vi "Test_PreloadNormalMsg_SendHighPriorityStop_StopImmediately.vi"(8 "error in (no error)":errorcluster, 11 "TestCase in":refnum<class "TestPriorityStopMessage.lvclass">) -> (0 "error out":errorcluster, 3 "TestCase out":refnum<class "TestPriorityStopMessage.lvclass">)   [LabVIEW 2017, in "TestPriorityStopMessage.lvclass"]
uses:
  TestPriorityStopMessage.lvclass
  <vilib>/ActorFramework/Message Enqueuer/Message Priority.ctl
  <vilib>/ActorFramework/Message Enqueuer/Message Enqueuer.lvclass/Message Enqueuer.ctl
  Doubles/MessageCountsExecutions/MessageCountsExecutions.lvclass
  C:/Program Files (x86)/National Instruments/LabVIEW 2017/vi.lib/ActorFramework/Message/Message.lvclass
  Doubles/ActorBlockedUntilNotified/ActorBlockedUntilNotified.lvclass
  C:/Program Files (x86)/National Instruments/LabVIEW 2017/vi.lib/ActorFramework/Actor/Actor.lvclass
  <vilib>/ActorFramework/Stop Msg/Stop Msg.lvclass
  <vilib>/ActorFramework/Message Priority Queue/Priority Enqueue.vi
  <vilib>/ActorFramework/Actor/Actor.lvclass
  <vilib>/ActorFramework/Message Enqueuer/Message Enqueuer.lvclass
  Source/PriorityStopMessage/PriorityStopMessage.lvclass
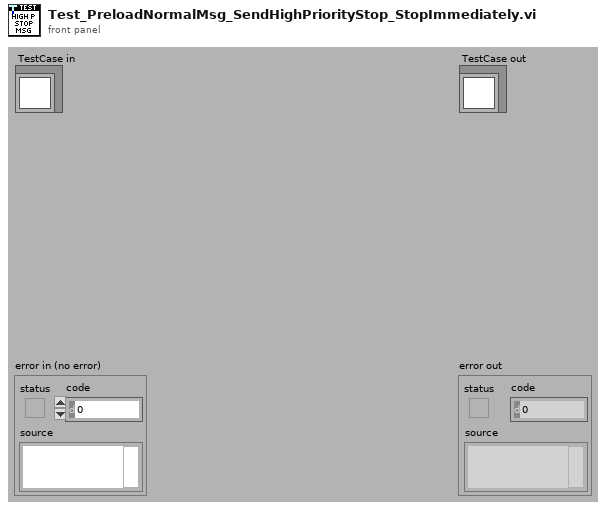
[diagram p1: front panel]
types:
  T1 = typedef "Actor Framework.lvlib/Message Enqueuer.lvclass/Message Priority.ctl" = enum16{"Low", "Normal", "High"}
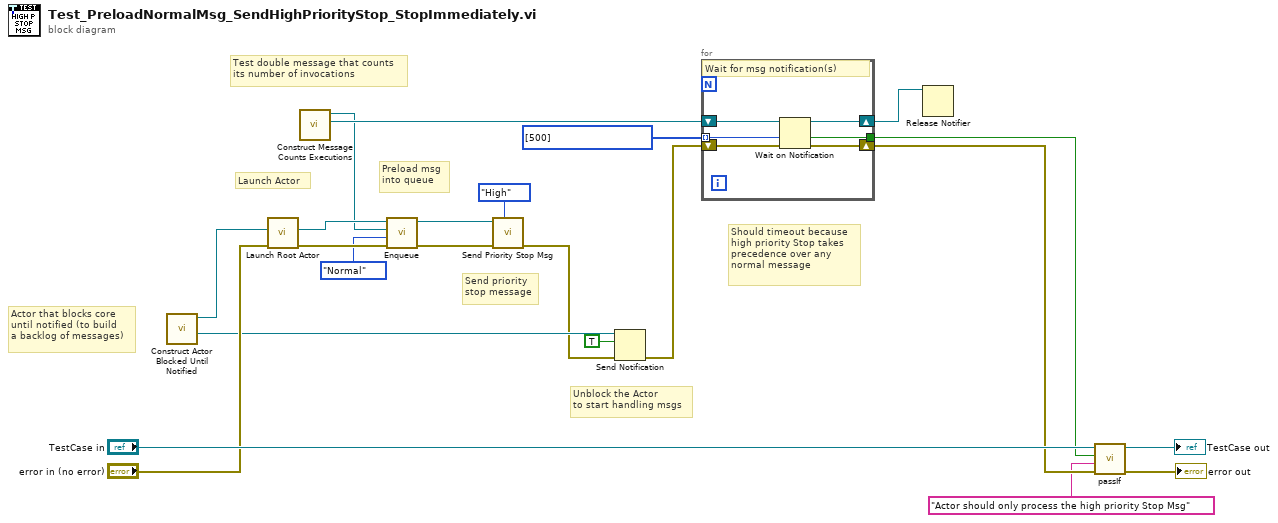
[diagram p0: block diagram]
diagram:
  # "Should timeout because\nhigh priority Stop takes\nprecedence over any\nnormal message"
  # "Send priority\nstop message"
  # "Preload msg\ninto queue"
  # "Unblock the Actor\nto start handling msgs"
  # "Actor that blocks core\nuntil notified (to build\na backlog of messages)"
  # "Test double message that counts\nits number of invocations"
  # "Launch Actor"
  n1 = call "Construct Actor Blocked Until Notified.vi"() -> ("Unblock Notifier"=w13:refnum<notifier>, "ActorBlockedUntilNotified"=w14:refnum<class "ActorBlockedUntilNotified.lvclass">)  [unwired: 10 in]
  n2 = call <vilib>:"Launch Root Actor.vi"("error in (no error)"="error in (no error)", "Actor"=w14) -> ("error out"=w17:errorcluster, "Actor's Enqueuer"=w10:refnum<class "Message Enqueuer.lvclass">)  [unwired: 8 in]
  n3 = call "Construct Message Counts Executions.vi"() -> ("Message Executions"=w18:refnum<notifier>, "CyclicMessageCountsCycles out"=w9:refnum<class "MessageCountsExecutions.lvclass">)  [unwired: 9 in, 1 out]
  n4 = call <vilib>:"Enqueue.vi"("error in (no error)"=w17, "Message Priority (Normal)"=Message_Priority."Normal" ("Message Priority"), "Message"=w9, "Message Enqueuer in"=w10) -> ("error out"=w11:errorcluster, "Message Enqueuer out"=w6:refnum<class "Message Enqueuer.lvclass">)  [unwired: 6 in]
  n5 = call "Send Priority Stop Msg.vi"("Message Priority (Normal)"=Message_Priority."High", "error in (no error)"=w11, "Message Enqueuer"=w6) -> ("error out"=w7:errorcluster)  [unwired: 8 in]
  n6 = Send Notification(notification=TRUE, notifier=w13, error in (no error)=w7) -> (error out=w5:errorcluster)  [unwired: 1 out]
  n7 = for {
    shift-right: [w27] -> w3
    shift-left: w18 -> [w28]
    shift-right: [w25] -> w16
    shift-left: w5 -> [w26]
    tunnel: [w24] -> w4
    tunnel: i32[] [500] -> [w23] mode=indexing
    # "Wait for msg notification(s)"
    n8 = Wait on Notification(notifier=w28, timeout in ms (-1)=w23, error in (no error)=w26) -> (notifier out=w27:refnum<notifier>, timed out?=w24:bool, error out=w25:errorcluster)  [unwired: 1 in, 1 out]
  }
  n9 = Release Notifier(notifier=w3) -> ()  [unwired: 2 in, 3 out]
  n10 = call-dynamic "passIf.vi"("error in (no error)"=w16, "message (\"\")"="Actor should only process the high priority Stop Msg" ("message (\"\")"), "pass"=w4, "TestCase in"="TestCase in") -> ("error out"=→"error out":errorcluster, "TestCase out"=→"TestCase out":refnum<class "TestPriorityStopMessage.lvclass">)  [unwired: 6 in]
